vi "(SubVI)System Command_Get Board Information.vi"(8 "error in (no error)":errorcluster caption="에러 입력(에러 없음)", 10 "ID to Exclude":u8 format="%.0x", 11 "ID to Find":u8 format="%.0x") -> (0 "error out":errorcluster caption="에러 출력", 1 "I2C Slave ID":cluster{string, u8}[](array[cluster]), 2 "BD HW Version":T2(ring), 3 "BD FW Version":u32 format="%08x", 4 "Default I2C Slave ID":u8, 5 "BD SN":string, 6 "IC Type":T1, 7 "BD Info Str":string)   [LabVIEW 2020]
uses:
  Libraries/Haptic IC Class/Haptic IC/Controls/(Ctrl)IC Type.ctl
  Serial/Controls/(Ctrl)Serial_Write Read Option.ctl
  Variables/(Var)System Variables.vi
  76a10119-0002-4f08-a14c-cf884ba6b7fd.vi
  Libraries/Haptic IC Class/Haptic IC/Haptic IC.lvclass
panel:
  # "(SubVI)System Command_Get Board Information.vi By hspark\n\nDescription : Board Information 요청 명령어를 보내 Board 정보를 읽는 VI\n\nInput : \n1. ID to Find : 9786 등과 같이 Chip ID 확인이 불가능한 IC의 경우, 찾으려는 ID를 입력받아서 ID List에 있는 경우 해당 ID가 선택되게 함\n\nOutput : \n1. BD FW Version : U32로 된 Board의 FW Version\n2. BD HW Version : 프로토콜에 명시된 Board의 HW Version (모델 추가 시 열거형 타입 정의 업데이트)\n3. I2C Slave ID : Board로부터 수신받은 I2C Slave ID 목록. 링 컨트롤 업데이트를 위한 클러스터 배열 출력.\n4. Default I2C Slave ID : Chip ID가 있는 첫번째 Slave ID. 모든 Slave가 Chip ID가 없는 경우 첫번째 Slave ID\n\nLabVIEW Version : 2020 SP1 이상\n\nNote :\nChip ID가 0x0020 인 경우만 케이스 처리하였음. (DW9781)\n다른 Chip에 대한 케이스 추가 필요\n\nUpdate : 2021.12.20"
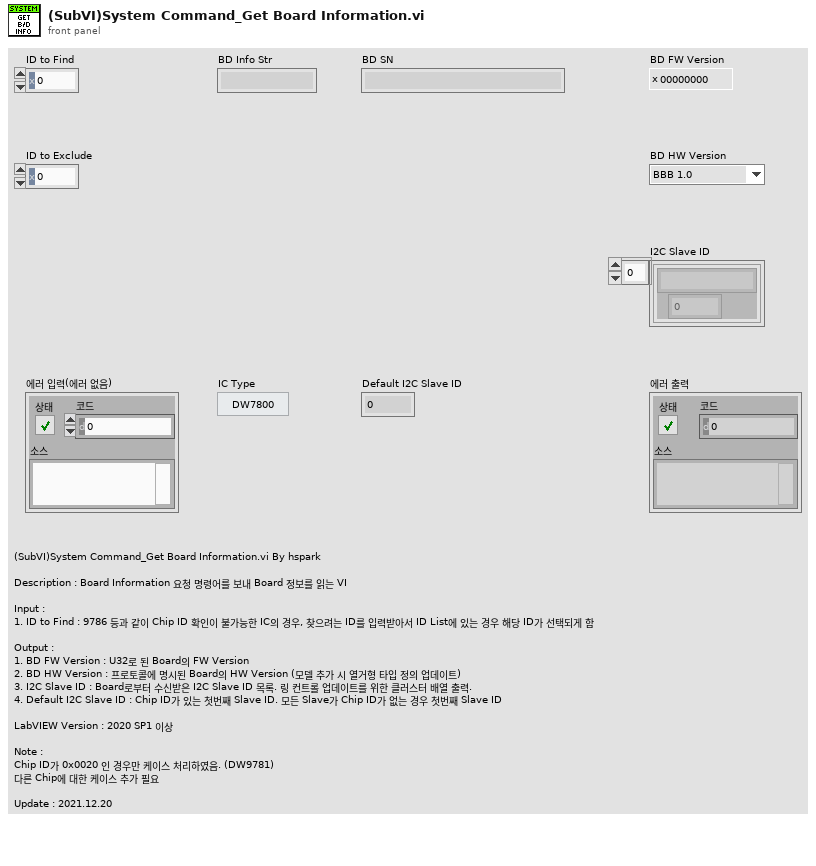
[diagram p1: front panel]
types:
  T1 = typedef "Haptic IC.lvclass/(Ctrl)IC Type.ctl" = enum8{"DW7800", "DW7802", "DW7912", "DW7914"}
  T2 = enum8{"BBB 1.0", "BBB 1.1", "WBB 1.0", "reserved", "RedNoah3"}
  T3 = typedef "(Ctrl)Serial_Write Read Option.ctl" = cluster{"Echo Request":bool, "Header Verification":bool, "Checksum Verification":bool, "User Code Verifiaction":bool}
  T4 = typedef "(Ctrl)Serial_Protocol Header.ctl" = cluster{"Delimiter Code":u8, "BD Info":u8, "Msg Size":u16, "Checksum":u8, "Echo Request":u8}
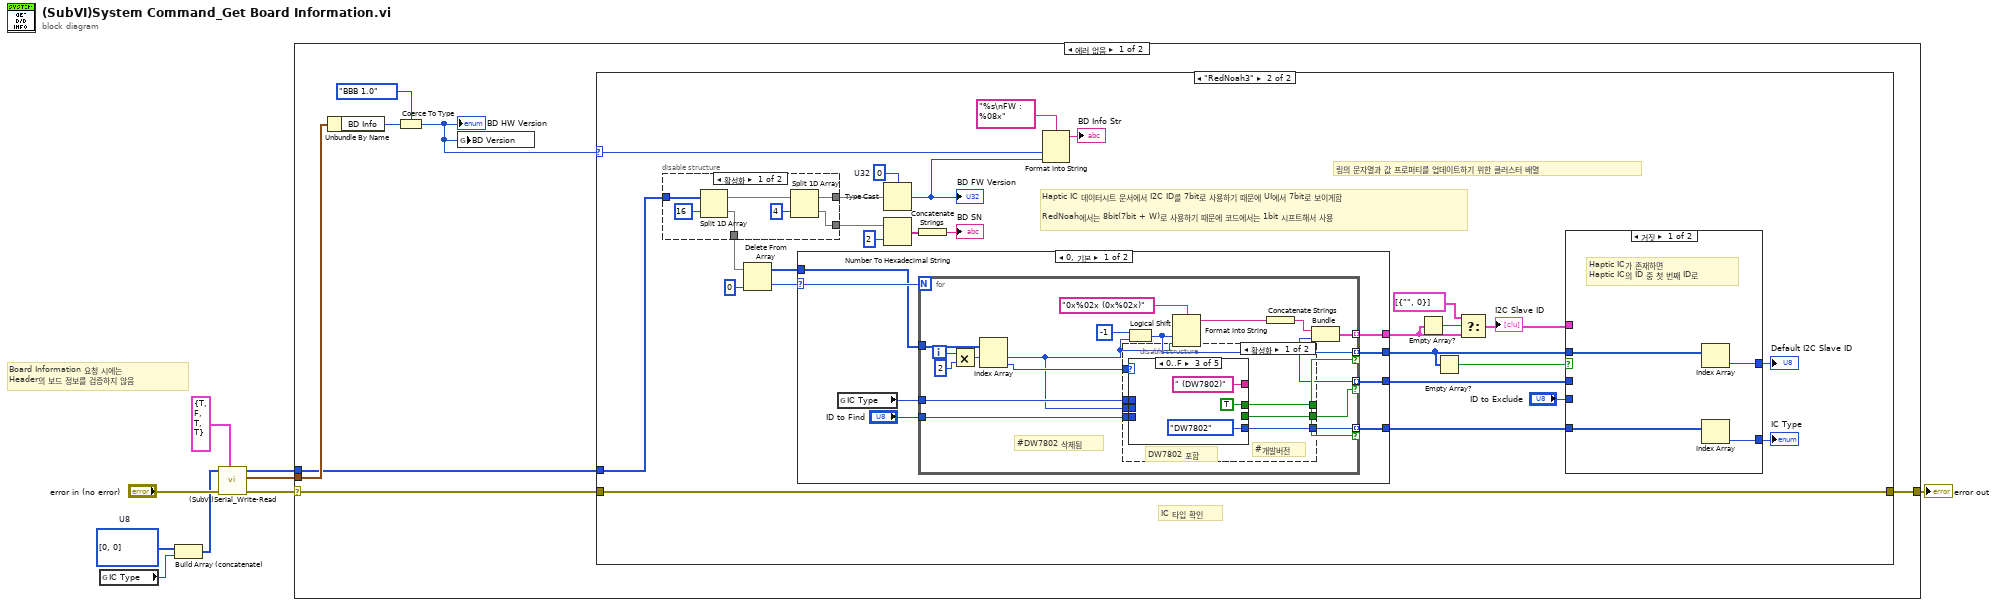
[diagram p0: block diagram]
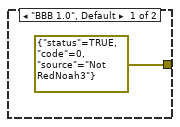
[diagram p2: hidden frame]
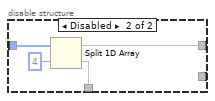
[diagram p3: hidden frame]
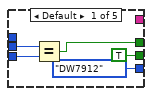
[diagram p4: hidden frame]
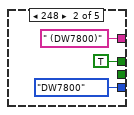
[diagram p5: hidden frame]
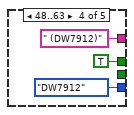
[diagram p6: hidden frame]
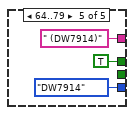
[diagram p7: hidden frame]
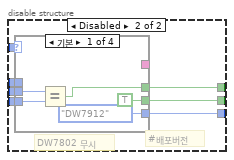
[diagram p8: hidden frame]
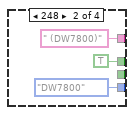
[diagram p9: hidden frame]
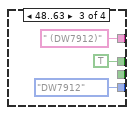
[diagram p10: hidden frame]
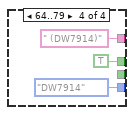
[diagram p11: hidden frame]
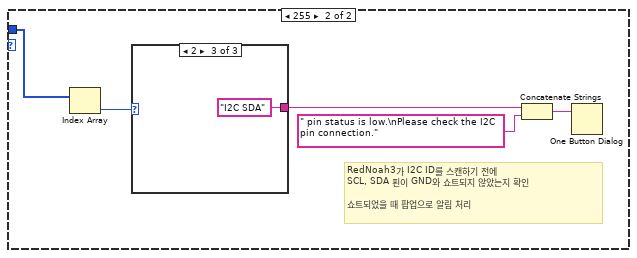
[diagram p12: hidden frame]
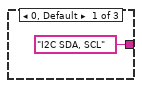
[diagram p13: hidden frame]
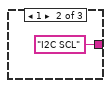
[diagram p14: hidden frame]
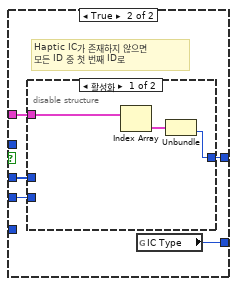
[diagram p15: hidden frame]
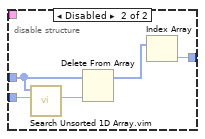
[diagram p16: hidden frame]
diagram:
  w3 = u8[] [0, 0]  # U8
  # "Board Information 요청 시에는\nHeader의 보드 정보를 검증하지 않음"
  n1 = global read "(Var)System Variables.vi" "IC Type"() -> (w2:T1)
  n2 = Build Array (concatenate)(w3, w2) -> (w1:u8[])
  n3 = call "(SubVI)Serial_Write-Read.vi"("Option"=T3 {"Echo Request"=TRUE, "Header Verification"=FALSE, "Checksum Verification"=TRUE, "User Code Verifiaction"=TRUE}, "error in (no error)"="error in (no error)", "Data to Write"=w1) -> ("error out"=w8:errorcluster, "Header"=w9:T4, "Read Data"=w6:u8[])  [unwired: 6 in]
  n4 = case shown="에러 없음" w8 {
    selector: w8 -> [w11 w151]
    tunnel: w9 -> [w16 _]
    tunnel: [w10 w151] -> w7
    tunnel: w6 -> [w15 _]
    frame No Error {
      n5 = Unbundle By Name(w16) -> ("BD Info"=w14:u8)
      n6 = Coerce To Type(0:w14, 1:T2."BBB 1.0" ("BD HW Version")) -> (2:w12:T2)
      "BD HW Version" <- w12
      n7 = global write "(Var)System Variables.vi" "BD Version"(w12) -> ()
      n8 = case shown="\"RedNoah3\"" w12 {
        selector: w12 -> [_ w33]
        tunnel: w15 -> [_ w37]
        tunnel: w11 -> [_ w18]
        tunnel: [errorcluster {"status"=TRUE, "code"=0, "source"="Not RedNoah3"} ("error IO") w18] -> w10
        frame "BBB 1.0", Default {
        }
        frame "RedNoah3" {
          w23 = u32 0  # U32
          # "IC 타입 확인"
          # "Haptic IC 데이터시트 문서에서 I2C ID를 7bit로 사용하기 때문에 UI에서 7bit로 보이게함\n\nRedNoah에서는 8bit(7bit + W)로 사용하기 때문에 코드에서는 1bit 시프트해서 사용"
          # "링의 문자열과 값 프로퍼티를 업데이트하기 위한 클러스터 배열"
          n9 = disable-structure shown="활성화" {
            disable-tunnel: [w49 w54] -> w44
            disable-tunnel: w37 -> [w48 w53]
            disable-tunnel: [w47 w52] -> w24
            disable-tunnel: [w45 _] -> w22
            frame Enabled {
              n10 = Split 1D Array(array=w48, index=16 ("인덱스")) -> (first subarray=w50:u8[], second subarray=w49:u8[])
              n11 = Split 1D Array(array=w50, index=4 ("인덱스")) -> (first subarray=w47:u8[], second subarray=w45:u8[])
            }
            frame Disabled {
              n12 = Split 1D Array(array=w53, index=4 ("인덱스")) -> (first subarray=w52:u8[], second subarray=w54:u8[])
            }
          }
          n13 = Delete From Array(array=w44, index=0 ("인덱스")) -> (deleted portion=w42:u8, array with subset deleted=w41:u8[])  [unwired: 1 in]
          n14 = case shown="0, 기본" w42 {
            selector: w42 -> [w63 _]
            tunnel: w41 -> [w62 w130]
            tunnel: [w61 _] -> w39
            tunnel: [w60 _] -> w27
            tunnel: [w57 _] -> w36
            tunnel: [w56 _] -> w30
            frame 0, Default {
              n15 = global read "(Var)System Variables.vi" "IC Type"() -> (w59:T1)
              n16 = for {
                N: w63 -> [_]
                tunnel: w62 -> [w80]
                tunnel: [w73] -> w60 mode=indexing
                tunnel: [w65] -> w61 mode=indexing if=w66
                tunnel: w59 -> [w72]
                tunnel: "ID to Find" -> [w71]
                tunnel: [w65] -> w57 mode=indexing if=w70
                tunnel: [w67] -> w56 mode=indexing if=w66
                i -> [w79]
                # "#DW7802 삭제됨"
                n17 = Multiply(x=w79, y=2) -> (x*y=w78:i32)
                n18 = Index Array(array=w80, index #1=w78) -> (element #1=w64:u8, element #2=w69:u8)  [unwired: 1 in]
                n19 = disable-structure shown="활성화" {
                  disable-tunnel: w72 -> [w87 w111]
                  disable-tunnel: w71 -> [w86 w110]
                  disable-tunnel: [w85 w109] -> w70
                  disable-tunnel: w69 -> [w84 w108]
                  disable-tunnel: [w83 w107] -> w67
                  disable-tunnel: [w82 w106] -> w66
                  disable-tunnel: w64 -> [w81 w105]
                  frame Enabled {
                    # "#개발버전"
                    # "DW7802 포함"
                    n20 = case shown="0..F" w84 {
                      tunnel: [_ " (DW7800)" " (DW7802)" " (DW7912)" " (DW7914)"] -> _
                      tunnel: [w90 TRUE TRUE TRUE TRUE] -> w82
                      tunnel: w87 -> [_ _ _ _ _]
                      tunnel: w81 -> [w92 _ _ _ _]
                      tunnel: w86 -> [w91 _ _ _ _]
                      tunnel: [TRUE _ _ _ _] -> w85
                      tunnel: [(Ctrl)IC_Type."DW7912" ("IC Type") (Ctrl)IC_Type."DW7800" ("IC Type") (Ctrl)IC_Type."DW7802" ("IC Type") (Ctrl)IC_Type."DW7912" ("IC Type") (Ctrl)IC_Type."DW7914" ("IC Type")] -> w83
                      frame Default {
                        n21 = Equal?(x=w92, y=w91) -> (x = y?=w90:bool)
                      }
                      frame 248 {
                      }
                      frame 0..15 {
                      }
                      frame 48..63 {
                      }
                      frame 64..79 {
                      }
                    }
                  }
                  frame Disabled {
                    # "#배포버전"
                    # "DW7802 무시"
                    n22 = case shown="기본" w108 {
                      tunnel: [_ " (DW7800)" " (DW7912)" " (DW7914)"] -> _
                      tunnel: [w114 TRUE TRUE TRUE] -> w106
                      tunnel: w111 -> [_ _ _ _]
                      tunnel: w105 -> [w116 _ _ _]
                      tunnel: w110 -> [w115 _ _ _]
                      tunnel: [TRUE _ _ _] -> w109
                      tunnel: [(Ctrl)IC_Type."DW7912" ("IC Type") (Ctrl)IC_Type."DW7800" ("IC Type") (Ctrl)IC_Type."DW7912" ("IC Type") (Ctrl)IC_Type."DW7914" ("IC Type")] -> w107
                      frame Default {
                        n23 = Equal?(x=w116, y=w115) -> (x = y?=w114:bool)
                      }
                      frame 248 {
                      }
                      frame 48..63 {
                      }
                      frame 64..79 {
                      }
                    }
                  }
                }
                n24 = Logical Shift(y=i16 -1, x=w64) -> (x << y=w65:u8)
                n25 = Format Into String(format string="0x%02x (0x%02x)" ("포맷 문자열"), w65, w64) -> (resulting string=w75:string)  [unwired: 2 in, 1 out]
                n26 = Concatenate Strings(w75) -> (w74:string)
                n27 = Bundle(w74, w65) -> (w73:cluster{string, u8})  [unwired: 1 in]
              }
            }
            frame 255 {
              # "RedNoah3가 I2C ID를 스캔하기 전에\nSCL, SDA 핀이 GND와 쇼트되지 않았는지 확인\n\n쇼트되었을 때 팝업으로 알림 처리"
              n28 = Index Array(array=w130) -> (element=w129:u8)  [unwired: 1 in]
              n29 = case shown="2" w129 {
                tunnel: ["I2C SDA, SCL" "I2C SCL" "I2C SDA"] -> w127
                frame 0, Default {
                }
                frame 1 {
                }
                frame 2 {
                }
              }
              n30 = Concatenate Strings(w127, " pin status is low.\nPlease check the I2C pin connection." ("문자열")) -> (w128:string)
              n31 = One Button Dialog(message=w128) -> ()  [unwired: 1 in, 1 out]
            }
          }
          n32 = Type Cast(type=w23, x=w24) -> (*(type *) &x=w32:u32)
          "BD FW Version" <- w32
          n33 = Number To Hexadecimal String(1:i16 2 ("폭(-)"), 2:w22) -> (0:w20:string[])
          n34 = Concatenate Strings(w20) -> (→"BD SN":string)
          n35 = Format Into String(format string="%s\nFW : %08x" ("포맷 문자열"), w33, w32) -> (resulting string=→"BD Info Str":string)  [unwired: 2 in, 1 out]
          n36 = Empty Array?(array=w27) -> (empty?=w28:bool)
          n37 = Empty Array?(array=w39) -> (empty?=w40:bool)
          n38 = Select(t=cluster{string, u8}[] [{"", 0}], s=w28, f=w27) -> (s? t:f=w26:cluster{string, u8}[])
          "I2C Slave ID" <- w26
          n39 = case shown="거짓" w40 {
            tunnel: w39 -> [w137 _]
            tunnel: w26 -> [_ w142]
            tunnel: [w136 w141] -> w38
            tunnel: w36 -> [_ w140]
            tunnel: "ID to Exclude" -> [_ w139]
            tunnel: w30 -> [w135 _]
            tunnel: [w134 w138] -> w29
            frame False {
              # "Haptic IC가 존재하면\nHaptic IC의 ID 중 첫 번째 ID로"
              n40 = Index Array(array=w137) -> (element=w136:u8)  [unwired: 1 in]
              n41 = Index Array(array=w135) -> (element=w134:T1)  [unwired: 1 in]
            }
            frame True {
              # "Haptic IC가 존재하지 않으면\n모든 ID 중 첫 번째 ID로"
              n42 = disable-structure shown="활성화" {
                disable-tunnel: w142 -> [w145 _]
                disable-tunnel: [w143 w150] -> w141
                disable-tunnel: w140 -> [_ w149]
                disable-tunnel: w139 -> [_ w148]
                frame Enabled {
                  n43 = Index Array(array=w145) -> (element=w144:cluster{string, u8})  [unwired: 1 in]
                  n44 = Unbundle(w144) -> (w143:u8)  [unwired: 1 out]
                }
                frame Disabled {
                  n45 = call "Search Unsorted 1D Array.vim"("element"=w148, "unsorted 1D array"=w149) -> ("index of element"=w146:i32)  [unwired: 9 in]
                  n46 = Delete From Array(array=w149, index=w146) -> (array with subset deleted=w147:u8[])  [unwired: 1 in, 1 out]
                  n47 = Index Array(array=w147) -> (element=w150:u8)  [unwired: 1 in]
                }
              }
              n48 = global read "(Var)System Variables.vi" "IC Type"() -> (w138:T1)
            }
          }
          "Default I2C Slave ID" <- w38
          "IC Type" <- w29
        }
      }
    }
    frame Error {
    }
  }
  "error out" <- w7
